vi "AutoShoot.vi"(9 "Reset?":bool, 11 "Array":dbl[](array[numeric]) format="%0.3f") -> (3 "isFinished":bool)   [LabVIEW 2013]
uses:
  Shooter/Shooter Command.ctl
  Shooter/Shooter Manual Control.ctl
  Robot Global Data.vi
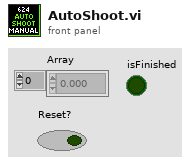
[diagram p1: front panel]
types:
  T1 = typedef "Shooter Manual Control.ctl" = cluster{"Command":T2, "Offset":dbl, "Trigger":bool, "Add":bool, "Release":bool, "Reset":bool, "Target Pressure":dbl, "Punch":bool, "AutoPunch":bool}
  T2 = typedef "Shooter Command.ctl" = enum16{"None", "Warmup", "Shoot", "Line Shoot", "Soft Shoot", "Toss"}
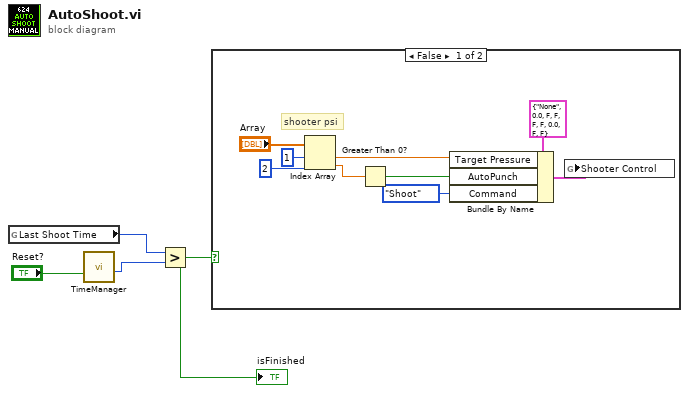
[diagram p0: block diagram]
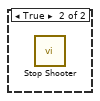
[diagram p2: hidden frame]
diagram:
  n1 = global read "Robot Global Data.vi" "Last Shoot Time"() -> (w3:u32)
  n2 = call "TimeManager.vi"("Reset?"="Reset?") -> ("Start Time"=w2:u32)  [unwired: 9 in, 1 out]
  n3 = Greater?(x=w3, y=w2) -> (0:w1:bool)
  "isFinished" <- w1
  n4 = case shown="False" w1 {
    frame False {
      # "shooter psi"
      n5 = Index Array(array="Array", index #1=1 ("index"), index #2=2 ("index")) -> (element #1=w8:dbl, element #2=w7:dbl)
      n6 = Greater Than 0?(x=w7) -> (x > 0?=w6:bool)
      n7 = Bundle By Name(cluster=T1 {"Command"=enum."None", "Offset"=0.0, "Trigger"=FALSE, "Add"=FALSE, "Release"=FALSE, "Reset"=FALSE, "Target Pressure"=0.0, "Punch"=FALSE, "AutoPunch"=FALSE} ("Shooter Manual Control"), "Target Pressure"=w8, "AutoPunch"=w6, "Command"=Shooter_Command."Shoot" ("Enum")) -> (w10:T1)
      n8 = global write "Robot Global Data.vi" "Shooter Control"(w10) -> ()
    }
    frame True {
      n9 = call "Stop Shooter.vi"() -> ()  [unwired: 12 in]
    }
  }
